vi "Autonomous Independent.vi"   [LabVIEW 2012]
doc: "This VI is called when autonomous begins, and will automatically be terminated when autonomous ends. You can carry out timed or sensor driven robot movement independently without needing to return to the caller."
uses:
  Robot Global Data.vi
panel:
  # "Be sure to right-click and choose Data Operations>>Make Current Value default if you want to save the array values with the VI"
types:
  T1 = typedef "WPI_JoystickDevRef.ctl" = cluster{"Device":T2}
  T2 = typedef "WPI_JoystickDeviceEnum.ctl" = enum16{"USB 1", "USB 2", "USB 3", "USB 4", "Kinect 1", "Kinect 2"}
  T3 = cluster{"axis 1 (x)":dbl, "axis 2 (y)":dbl, "axis 3 (throttle)":dbl, "axis 4":dbl, "axis 5":dbl, "axis 6":dbl}
  T4 = typedef "WPI_MotorControlDeviceRef.ctl" = cluster{"DeviceStatus":errorcluster, "Type":enum16{"PWM", "CAN"}, "PWM":cluster{"Digital Module":T5, "PWM Channel":T6, "DeadBand":T7}, "CAN":cluster{"Device Number":u8, "Control Mode":T8, "Semaphore":T9, "Max Vout":dbl}, "Invert":bool, "TransformRef":T10, "InvTransformRef":T10}
  T5 = typedef "FPGA_TypedefDigitalModule.ctl" = enum16{"Digital Module 1", "Digital Module 2"}
  T6 = typedef "FPGA_DIOPWMChannel.ctl" = enum8{"PWM 1", "PWM 2", "PWM 3", "PWM 4", "PWM 5", "PWM 6", "PWM 7", "PWM 8", "PWM 9", "PWM 10", "Invalid"}
  T7 = typedef "WPI_PWMDeadband.ctl" = cluster{"Name":string, "maxPositivePwm":i32, "minPositivePwm":i32, "centerPwm":i32, "maxNegativePwm":i32, "minNegativePwm":i32, "angularRange":u16}
  T8 = typedef "WPI_CANJaguar_ControlMode.ctl" = enum8{"Percent VBus", "Current", "Speed", "Position", "Voltage"}
  T9 = typedef "Semaphore RefNum" = refnum<k1>
  T10 = typedef "WPI_PWMTransform_ConPane.ctl" = refnum<vi>
  T11 = typedef "WPI_AnalogChannelDevRef.ctl" = cluster{"DevStatus":errorcluster, "Analog Module":T12, "Analog Channel":T13}
  T12 = typedef "FPGA_TypedefAnalogModule.ctl" = enum16{"Analog Module 1", "Analog Module 2"}
  T13 = typedef "FPGA_AIChannel.ctl" = enum8{"AI 1", "AI 2", "AI 3", "AI 4", "AI 5", "AI 6", "AI 7", "AI 8", "Invalid"}
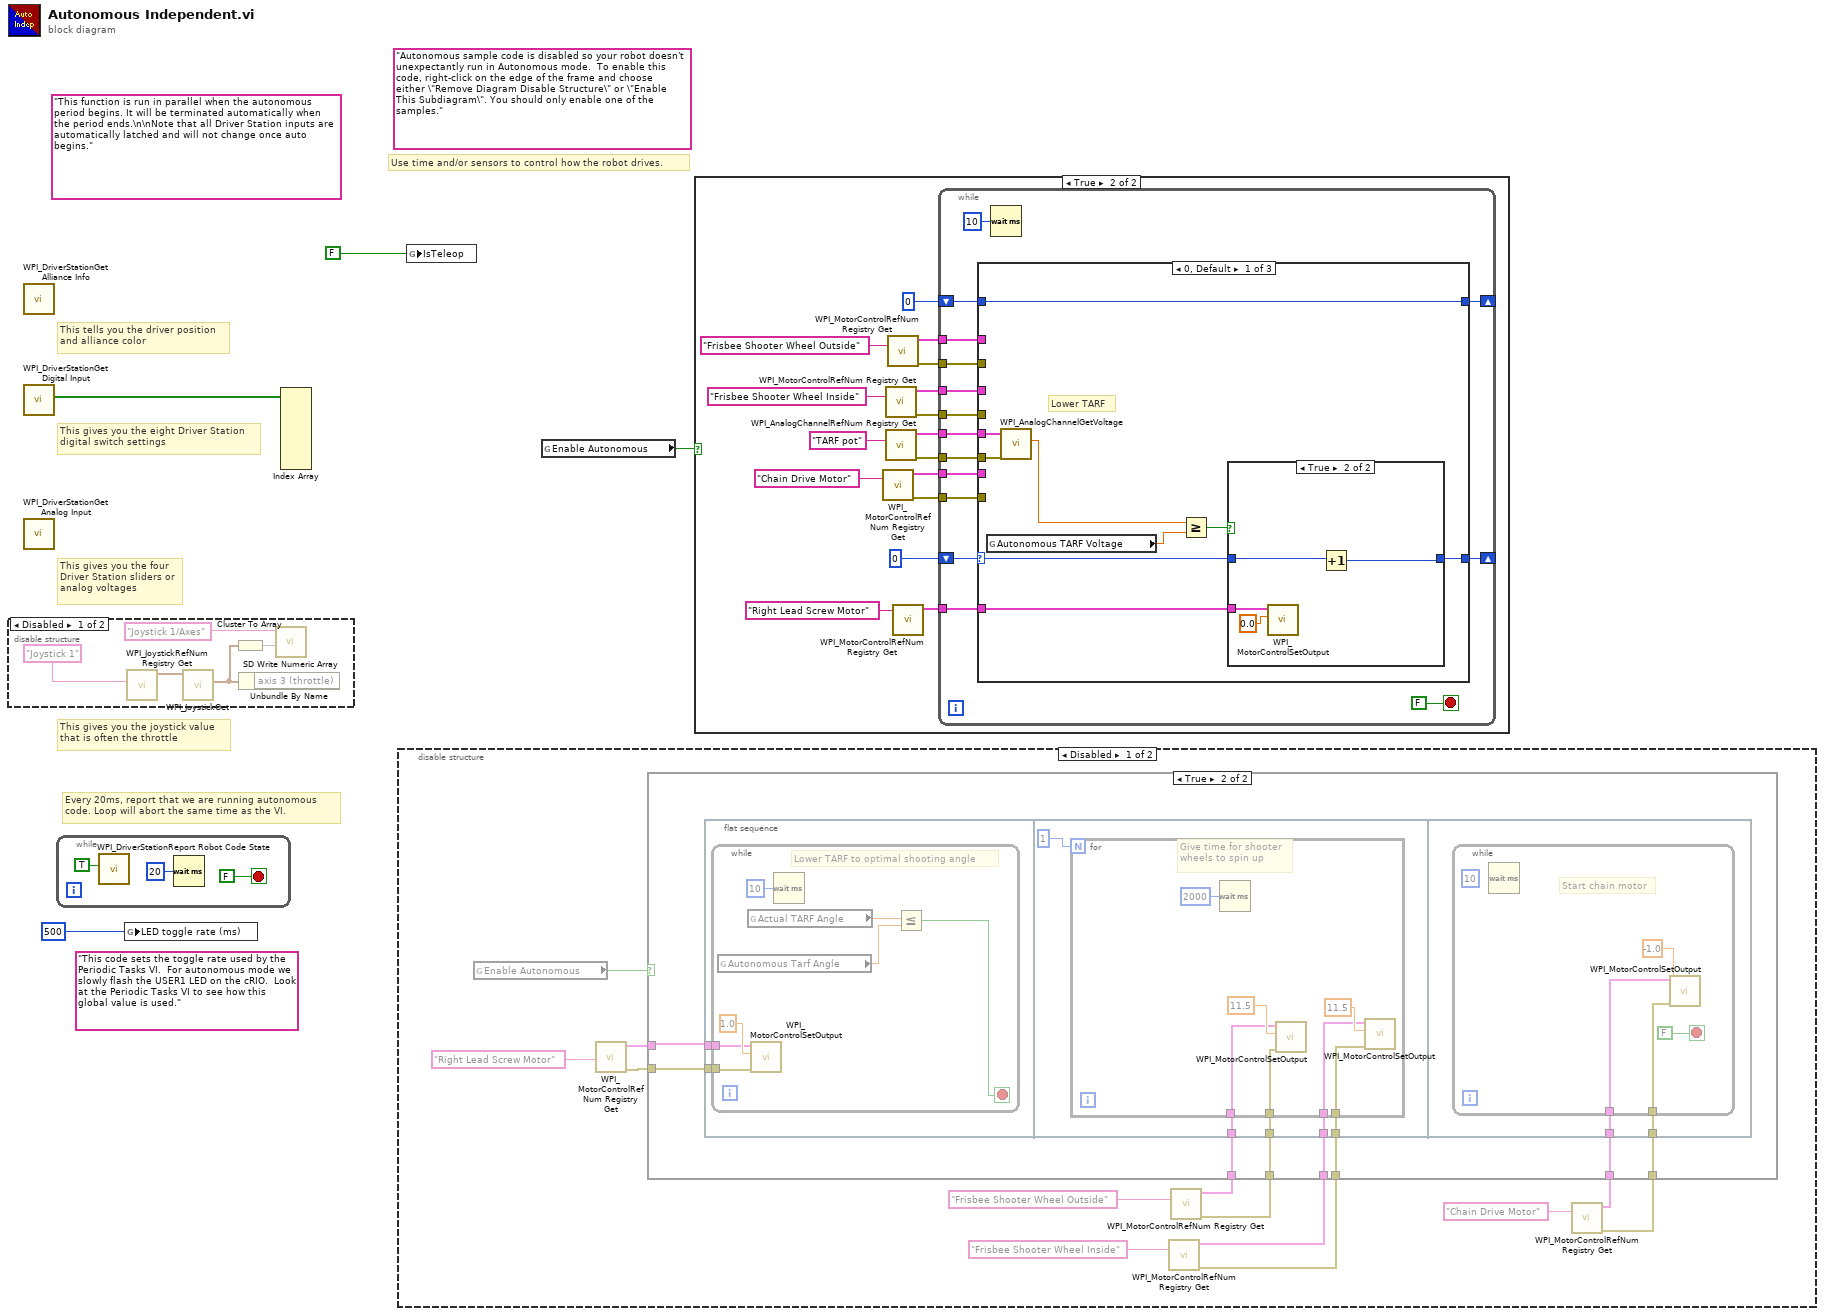
[diagram p0: block diagram]
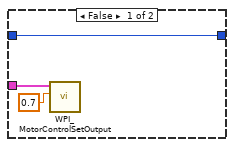
[diagram p3: hidden frame]
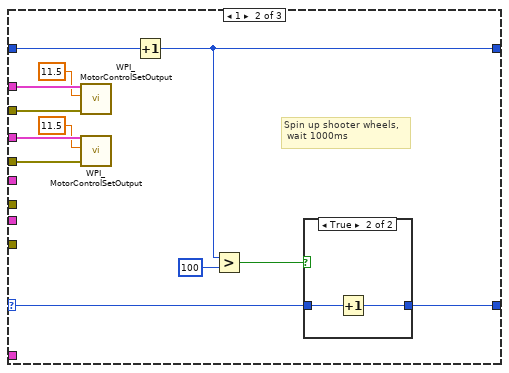
[diagram p4: hidden frame]
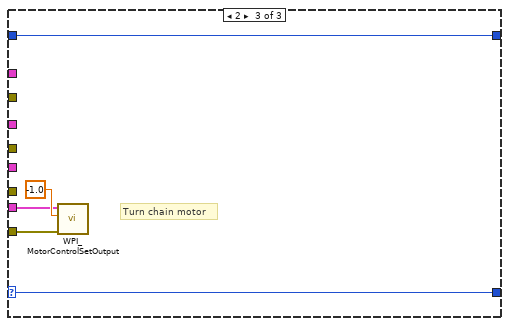
[diagram p6: hidden frame]
diagram:
  (unwired) "Autonomous sample code is disabled so your robot doesn't unexpectantly run in Autonomous mode.  To enable this code, right-click on the edge of the frame and choose either \"Remove Diagram Disable Structure\" or \"Enable This Subdiagram\". You should only enable one of the samples."
  (unwired) "This code sets the toggle rate used by the Periodic Tasks VI.  For autonomous mode we slowly flash the USER1 LED on the cRIO.  Look at the Periodic Tasks VI to see how this global value is used."
  (unwired) "This function is run in parallel when the autonomous period begins. It will be terminated automatically when the period ends.\n\nNote that all Driver Station inputs are automatically latched and will not change once auto begins."
  # "Use time and/or sensors to control how the robot drives."
  # "This tells you the driver position\nand alliance color"
  # "This gives you the eight Driver Station\ndigital switch settings"
  # "Every 20ms, report that we are running autonomous\ncode. Loop will abort the same time as the VI."
  # "This gives you the joystick value\nthat is often the throttle"
  # "This gives you the four\nDriver Station sliders or\nanalog voltages"
  n1 = disable-structure shown="Disabled" {
    frame Disabled {
      n2 = call <vilib>:"WPI_JoystickRefNum Registry Get.vi"("refnum name"="Joystick 1") -> ("JoystickDevRef"=w8:T1)  [unwired: 1 in, 9 out]
      n3 = call <vilib>:"WPI_JoystickGet.vi"("JoystickDevRef"=w8) -> ("Axes"=w6:T3)  [unwired: 1 in, 5 out]
      n4 = Cluster To Array(cluster=w6) -> (array=w7:dbl[])
      n5 = Unbundle By Name(w6) -> ()  [unwired: 1 out]
      n6 = call <vilib>:"SD Write Numeric Array.vi"("Numeric Array"=w7, "Name"="Joystick 1/Axes") -> ()  [unwired: 8 in, 2 out]
    }
    frame Enabled {
    }
  }
  n7 = call <vilib>:"WPI_DriverStationGet Alliance Info.vi"() -> ()  [unwired: 12 out]
  n8 = call <vilib>:"WPI_DriverStationGet Digital Input.vi"() -> ("Driver Station Digital Input (1-8)"=w4:bool[])  [unwired: 11 out]
  n9 = call <vilib>:"WPI_DriverStationGet Analog Input.vi"() -> ()  [unwired: 12 out]
  n10 = while {
    stop <- FALSE stop-if-true
    n11 = call <vilib>:"WPI_DriverStationReport Robot Code State.vi"("Autonomous"=TRUE) -> ()  [unwired: 10 in, 1 out]
    n12 = Wait (ms)(milliseconds to wait=u32 20) -> ()  [unwired: 1 out]
  }
  n13 = global write "Robot Global Data.vi" "LED toggle rate (ms)"(u32 500 ("LED ms toggle rate")) -> ()
  n14 = Index Array(array=w4) -> ()  [unwired: 8 in, 8 out]
  n15 = disable-structure shown="Disabled" {
    frame Disabled {
      n16 = global read "Robot Global Data.vi" "Enable Autonomous"() -> (w25:bool)
      n17 = call <vilib>:"WPI_MotorControlRefNum Registry Get.vi"("refnum name"="Right Lead Screw Motor") -> ("error out"=w22:errorcluster, "MotorControlDevRef"=w23:T4)  [unwired: 9 in]
      n18 = call <vilib>:"WPI_MotorControlRefNum Registry Get.vi"("refnum name"="Frisbee Shooter Wheel Inside") -> ("error out"=w13:errorcluster, "MotorControlDevRef"=w20:T4)  [unwired: 9 in]
      n19 = call <vilib>:"WPI_MotorControlRefNum Registry Get.vi"("refnum name"="Frisbee Shooter Wheel Outside") -> ("error out"=w14:errorcluster, "MotorControlDevRef"=w18:T4)  [unwired: 9 in]
      n20 = call <vilib>:"WPI_MotorControlRefNum Registry Get.vi"("refnum name"="Chain Drive Motor") -> ("error out"=w15:errorcluster, "MotorControlDevRef"=w16:T4)  [unwired: 9 in]
      n21 = case shown="True" w25 {
        tunnel: w23 -> [_ w33]
        tunnel: w22 -> [_ w32]
        tunnel: w20 -> [_ w31]
        tunnel: w18 -> [_ w30]
        tunnel: w16 -> [_ w29]
        tunnel: w15 -> [_ w28]
        tunnel: w14 -> [_ w27]
        tunnel: w13 -> [_ w26]
        frame False {
        }
        frame True {
          n22 = flat-sequence {
            tunnel: w33 -> [w35]
            tunnel: w32 -> [w34]
            tunnel: w31 -> [w46]
            tunnel: w30 -> [w45]
            tunnel: w27 -> [w44]
            tunnel: w26 -> [w43]
            tunnel: w29 -> [w56]
            tunnel: w28 -> [w55]
            frame #0 {
              n23 = while {
                tunnel: w35 -> [w37]
                tunnel: w34 -> [w36]
                stop <- w40 stop-if-true
                # "Lower TARF to optimal shooting angle"
                n24 = global read "Robot Global Data.vi" "Autonomous Tarf Angle"() -> (w41:dbl)
                n25 = global read "Robot Global Data.vi" "Actual TARF Angle"() -> (w42:dbl)
                n26 = call <vilib>:"WPI_MotorControlSetOutput.vi"("error in (no error)"=w36, "Output"=1.0, "MotorControlDevRef"=w37) -> ()  [unwired: 6 in, 3 out]
                n27 = Wait (ms)(milliseconds to wait=u32 10) -> ()  [unwired: 1 out]
                n28 = Less Or Equal?(x=w42, y=w41) -> (x <= y?=w40:bool)
              }
            }
            frame #1 {
              n29 = for {
                N: 1 -> [_]
                tunnel: w46 -> [w51]
                tunnel: w45 -> [w50]
                tunnel: w44 -> [w49]
                tunnel: w43 -> [w48]
                # "Give time for shooter\nwheels to spin up"
                n30 = Wait (ms)(milliseconds to wait=u32 2000) -> ()  [unwired: 1 out]
                n31 = call <vilib>:"WPI_MotorControlSetOutput.vi"("error in (no error)"=w49, "Output"=11.5, "MotorControlDevRef"=w50) -> ()  [unwired: 6 in, 3 out]
                n32 = call <vilib>:"WPI_MotorControlSetOutput.vi"("error in (no error)"=w48, "Output"=11.5, "MotorControlDevRef"=w51) -> ()  [unwired: 6 in, 3 out]
              }
            }
            frame #2 {
              n33 = while {
                tunnel: w56 -> [w58]
                tunnel: w55 -> [w57]
                stop <- FALSE stop-if-true
                (unwired) u32 10 ("milliseconds to wait")
                # "Start chain motor"
                n34 = Wait (ms)() -> ()  [unwired: 1 in, 1 out]
                n35 = call <vilib>:"WPI_MotorControlSetOutput.vi"("error in (no error)"=w57, "Output"=-1.0, "MotorControlDevRef"=w58) -> ()  [unwired: 6 in, 3 out]
              }
            }
          }
        }
      }
    }
    frame Enabled {
    }
  }
  n36 = global write "Robot Global Data.vi" "IsTeleop"(FALSE ("InTeleop")) -> ()
  n37 = global read "Robot Global Data.vi" "Enable Autonomous"() -> (w2:bool)
  n38 = case shown="True" w2 {
    frame False {
    }
    frame True {
      n39 = call <vilib>:"WPI_MotorControlRefNum Registry Get.vi"("refnum name"="Chain Drive Motor") -> ("error out"=w64:errorcluster, "MotorControlDevRef"=w65:T4)  [unwired: 9 in]
      n40 = call <vilib>:"WPI_MotorControlRefNum Registry Get.vi"("refnum name"="Frisbee Shooter Wheel Inside") -> ("error out"=w68:errorcluster, "MotorControlDevRef"=w70:T4)  [unwired: 9 in]
      n41 = call <vilib>:"WPI_AnalogChannelRefNum Registry Get.vi"("refnum name"="TARF pot") -> ("error out"=w61:errorcluster, "AIDeviceRef"=w62:T11)  [unwired: 9 in]
      n42 = call <vilib>:"WPI_MotorControlRefNum Registry Get.vi"("refnum name"="Frisbee Shooter Wheel Outside") -> ("error out"=w69:errorcluster, "MotorControlDevRef"=w71:T4)  [unwired: 9 in]
      n43 = call <vilib>:"WPI_MotorControlRefNum Registry Get.vi"("refnum name"="Right Lead Screw Motor") -> ("MotorControlDevRef"=w74:T4)  [unwired: 9 in, 1 out]
      n44 = while {
        shift-right: [w88] -> _
        shift-left: 0 -> [w90]
        tunnel: w74 -> [w89]
        tunnel: w71 -> [w86]
        tunnel: w70 -> [w85]
        tunnel: w69 -> [w84]
        tunnel: w68 -> [w83]
        shift-right: [w81] -> _
        shift-left: 0 -> [w82]
        tunnel: w65 -> [w80]
        tunnel: w64 -> [w79]
        tunnel: w62 -> [w78]
        tunnel: w61 -> [w77]
        stop <- FALSE stop-if-true
        n45 = case shown="0, Default" w90 {
          selector: w90 -> [w98 w109 w124]
          tunnel: w89 -> [w99 _ _]
          tunnel: [w97 w108 w124] -> w88
          tunnel: w86 -> [_ w119 _]
          tunnel: w85 -> [_ w118 _]
          tunnel: w84 -> [_ w117 _]
          tunnel: w83 -> [_ w116 _]
          tunnel: w82 -> [w96 w113 w123]
          tunnel: [w96 w112 w123] -> w81
          tunnel: w80 -> [_ _ w126]
          tunnel: w79 -> [_ _ w125]
          tunnel: w78 -> [w95 _ _]
          tunnel: w77 -> [w94 _ _]
          frame 0, Default {
            # "Lower TARF"
            n46 = global read "Robot Global Data.vi" "Autonomous TARF Voltage"() -> (w92:dbl)
            n47 = call <vilib>:"WPI_AnalogChannelGetVoltage.vi"("error in (no error)"=w94, "AIDeviceRef"=w95) -> ("Voltage"=w93:dbl)  [unwired: 7 in, 2 out]
            n48 = Greater Or Equal?(x=w93, y=w92) -> (x >= y?=w100:bool)
            n49 = case shown="True" w100 {
              tunnel: w99 -> [w103 w106]
              tunnel: w98 -> [w101 w105]
              tunnel: [w101 w104] -> w97
              frame False {
                n50 = call <vilib>:"WPI_MotorControlSetOutput.vi"("Output"=0.7, "MotorControlDevRef"=w103) -> ()  [unwired: 7 in, 3 out]
              }
              frame True {
                n51 = call <vilib>:"WPI_MotorControlSetOutput.vi"("Output"=0.0, "MotorControlDevRef"=w106) -> ()  [unwired: 7 in, 3 out]
                n52 = Increment(x=w105) -> (x+1=w104:i32)
              }
            }
          }
          frame 1 {
            # "Spin up shooter wheels,\n wait 1000ms"
            n53 = call <vilib>:"WPI_MotorControlSetOutput.vi"("error in (no error)"=w117, "Output"=11.5, "MotorControlDevRef"=w119) -> ()  [unwired: 6 in, 3 out]
            n54 = call <vilib>:"WPI_MotorControlSetOutput.vi"("error in (no error)"=w116, "Output"=11.5, "MotorControlDevRef"=w118) -> ()  [unwired: 6 in, 3 out]
            n55 = Increment(x=w113) -> (x+1=w112:i32)
            n56 = Greater?(x=w112, y=100) -> (0:w110:bool)
            n57 = case shown="True" w110 {
              tunnel: w109 -> [w120 w122]
              tunnel: [w120 w121] -> w108
              frame False {
              }
              frame True {
                n58 = Increment(x=w122) -> (x+1=w121:i32)
              }
            }
          }
          frame 2 {
            # "Turn chain motor"
            n59 = call <vilib>:"WPI_MotorControlSetOutput.vi"("error in (no error)"=w125, "Output"=-1.0, "MotorControlDevRef"=w126) -> ()  [unwired: 6 in, 3 out]
          }
        }
        n60 = Wait (ms)(milliseconds to wait=u32 10) -> ()  [unwired: 1 out]
      }
    }
  }
